vi "Channel Basics Lesson 3.vi"() -> ()   [LabVIEW 2019]
doc: "This VI demonstrates basic use of a Tag channel as a replacement for a global variable."
uses:
  subVIs/Demo Global.vi
  <extravilib>/ChannelInstances/Tag-i32/Instantiate.vi
  <extravilib>/ChannelInstances/Tag-i32/EndpointRead.vi
  <extravilib>/ChannelInstances/Tag-i32/Endpoint.vi
  <extravilib>/ChannelInstances/Tag-i32.lvlib
panel:
  in  "Tab Control":T1(tab)
  out "Reader B":i32(graph)
  in  "Stop Reader B":bool
  out "Writer B":i32(graph)
  in  "Stop Writer B":bool
  in  "Stop C":bool
  out "Writer C":i32(graph)
  out "Reader C":i32(graph)
  in  "Stop Reader A":bool
  out "Reader A":i32(graph)
  in  "Stop Writer A":bool
  out "Writer A":i32(graph)
  # "Overview: This VI demonstrates use of a Tag channel as a replacement for a global variable.\n\nInstructions:\n1. Open the block diagram. Review the lessons presented there.\n2. Run the VI to see that the behavior of the variable implementation (above) is the same as the Tag channel implementation (below in the first tab), but the Tag offers another option with the stop signal (below in the second tab)."
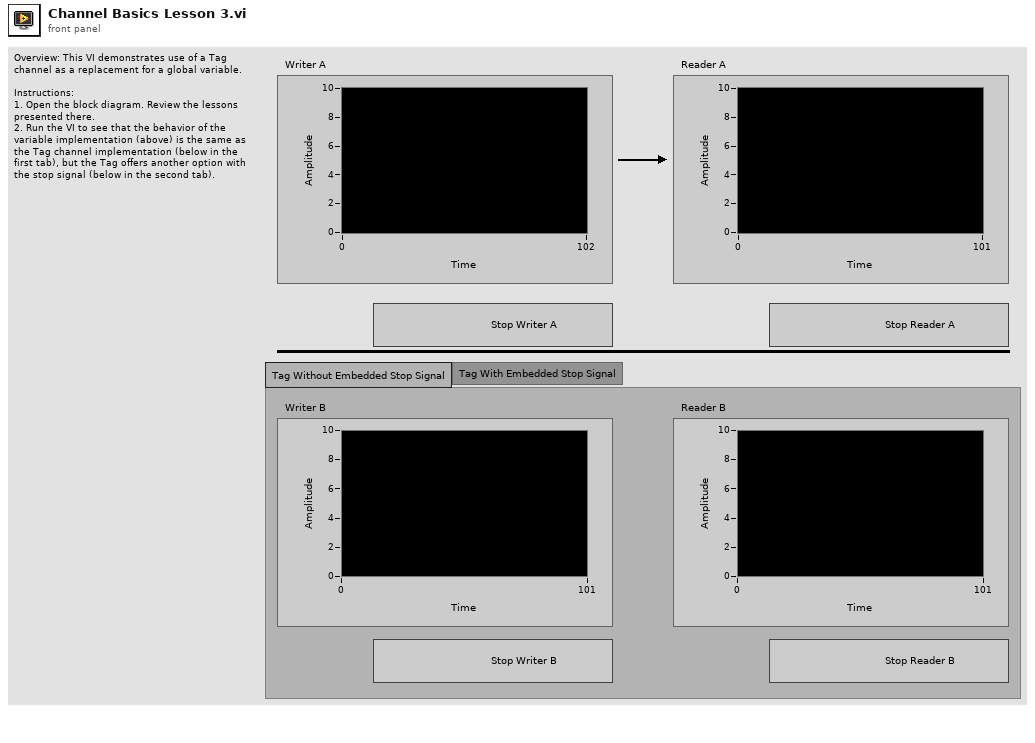
[diagram p1: front panel]
types:
  T1 = enum32{"Tag Without Embedded Stop Signal", "Tag With Embedded Stop Signal"}
  T2 = typedef "Tag-i32.lvlib/))Channel.ctl" = refnum<queue>
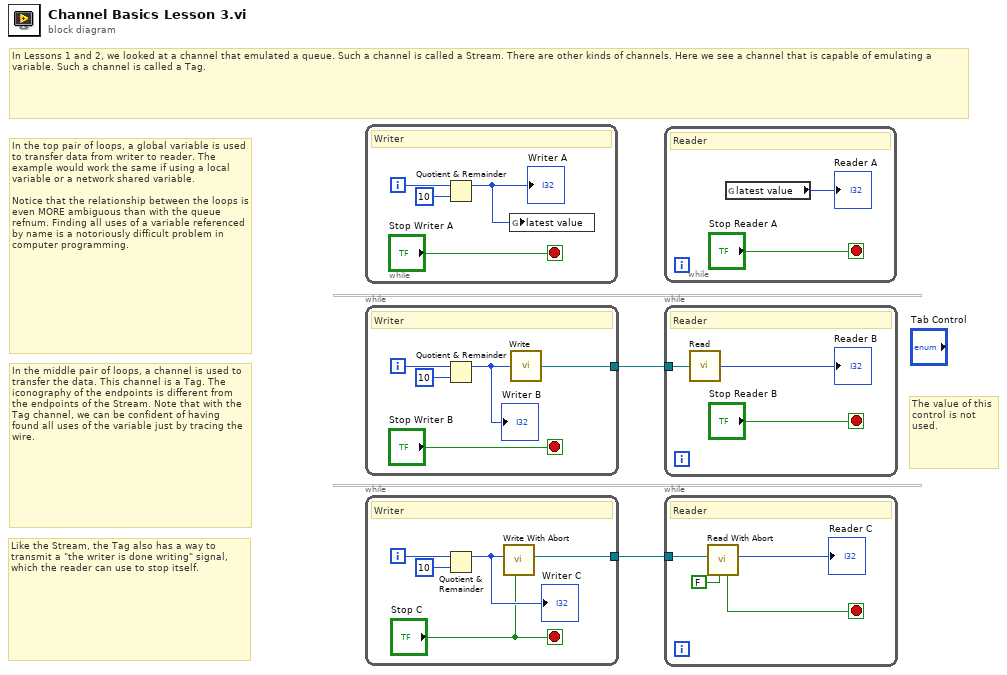
[diagram p0: block diagram]
diagram:
  # "The value of this control is not used."
  # "Like the Stream, the Tag also has a way to transmit a \"the writer is done writing\" signal, which the reader can use to stop itself."
  # "In the middle pair of loops, a channel is used to transfer the data. This channel is a Tag. The iconography of the endpoints is different from the endpoints of the Stream. Note that with the Tag channel, we can be confident of having found all uses of the variable just by tracing the wire."
  # "In the top pair of loops, a global variable is used to transfer data from writer to reader. The example would work the same if using a local variable or a network shared variable.\n\nNotice that the relationship between the loops is even MORE ambiguous than with the queue refnum. Finding all uses of a variable referenced by name is a notoriously difficult problem in computer programming."
  # "In Lessons 1 and 2, we looked at a channel that emulated a queue. Such a channel is called a Stream. There are other kinds of channels. Here we see a channel that is capable of emulating a variable. Such a channel is called a Tag."
  n1 = while {
    i -> [w5]
    stop <- "Stop Writer A" stop-if-true
    # "Writer"
    n2 = Quotient & Remainder(x=w5, y=10) -> (x-y*floor(x/y)=w3:i32)  [unwired: 1 out]
    "Writer A" <- w3
    n3 = global write "Demo Global.vi" "latest value"(w3) -> ()
  }
  n4 = while {
    tunnel: [w7] -> w2
    i -> [w10]
    stop <- "Stop Writer B" stop-if-true
    # "Writer"
    n5 = Quotient & Remainder(x=w10, y=10) -> (x-y*floor(x/y)=w8:i32)  [unwired: 1 out]
    "Writer B" <- w8
    n6 = call <extravilib>:"Write.vi"("element"=w8) -> ("channel"=w7:T2)  [unwired: 1 out]
  }
  n7 = while {
    tunnel: [w14] -> w1
    i -> [w15]
    stop <- "Stop C" stop-if-true
    # "Writer"
    n8 = Quotient & Remainder(x=w15, y=10) -> (x-y*floor(x/y)=w13:i32)  [unwired: 1 out]
    "Writer C" <- w13
    n9 = call <extravilib>:"Write With Abort.vi"("abort"="Stop C", "element"=w13) -> ("channel"=w14:T2)  [unwired: 7 in, 2 out]
  }
  n10 = while {
    stop <- "Stop Reader A" stop-if-true
    # "Reader"
    n11 = global read "Demo Global.vi" "latest value"() -> (→"Reader A":i32)
  }
  n12 = while {
    tunnel: w2 -> [w20]
    stop <- "Stop Reader B" stop-if-true
    # "Reader"
    n13 = call <extravilib>:"Read.vi"("channel"=w20) -> ("element"=→"Reader B":i32)  [unwired: 1 in, 1 out]
  }
  n14 = while {
    tunnel: w1 -> [w25]
    stop <- w23 stop-if-true
    # "Reader"
    n15 = call <extravilib>:"Read With Abort.vi"("abort"=FALSE, "channel"=w25) -> ("element"=→"Reader C":i32, "aborted?"=w23:bool)  [unwired: 7 in, 1 out]
  }
